vi "Tegam4040 -- GetDacValue.vi"(8 "error in (no error)":errorcluster, 11 "Instrument Session Handle In":u32 format="%x") -> (0 "error out":errorcluster, 2 "Dac Value":u16 format="%x", 3 "Instrument Session Handle Out (dupl)":u32 format="%x")   [LabVIEW 2010]
panel:
  out "VISA Error Code":i32 format="%x"
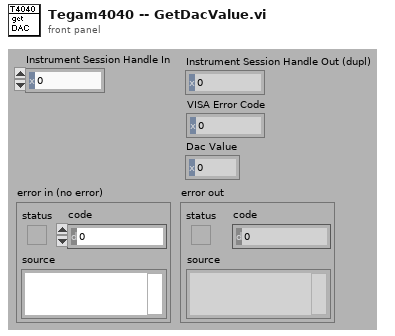
[diagram p1: front panel]
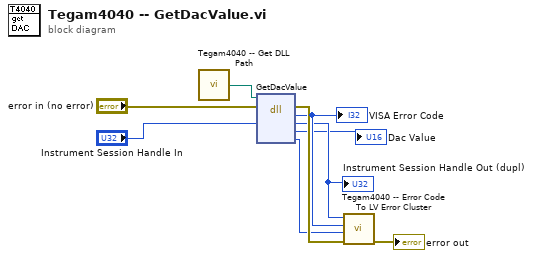
[diagram p0: block diagram]
diagram:
  n1 = call "Tegam4040 -- Get DLL Path.vi"() -> ("DLL Path"=w6:path)  [unwired: 8 in]
  n2 = dll-call lib="F:/My Documents/Code/Tegam4040CDriver/release/Tegam4040CDriver.dll" fn="GetDacValue" ("Tegam4040CDriver.dll:Close4040")(path in=w6, error in="error in (no error)", "instrSession"="Instrument Session Handle In") -> (error out=w8:errorcluster, "status"=w4:i32, "instrSession"=w3:u32, "dacValue"=→"Dac Value":u16, "driverError"=w2:i32)  [unwired: 3 in, 1 out]
  "VISA Error Code" <- w4
  "Instrument Session Handle Out (dupl)" <- w3
  n3 = call "Tegam4040 -- Error Code To LV Error Cluster.vi"("error in (no error)"=w8, "Driver Error Code"=w2, "VISA Error Code"=w4, "Instrument Session Handle"=w3) -> ("error out"=→"error out":errorcluster)  [unwired: 7 in]
